vi "Read.vi"(7 "Delay (On)":bool=TRUE caption="Delay(ON)", 8 "error in (no error)":errorcluster, 9 "Termination Character (10)":u8=10, 10 "Byte Count (1024)":u32=1024, 11 "VISA resource name":refnum<visa-resource-name>) -> (0 "error out":errorcluster, 1 "Return Count":u32, 2 "Read Buffer":string, 3 "VISA resource name out":refnum<visa-resource-name>)   [LabVIEW 2009, in "DSO1K.lvlib"]
doc: "Reads the returns the data in read buffer."
uses:
  <instrlib>/DSO1K/DSO1K.lvlib
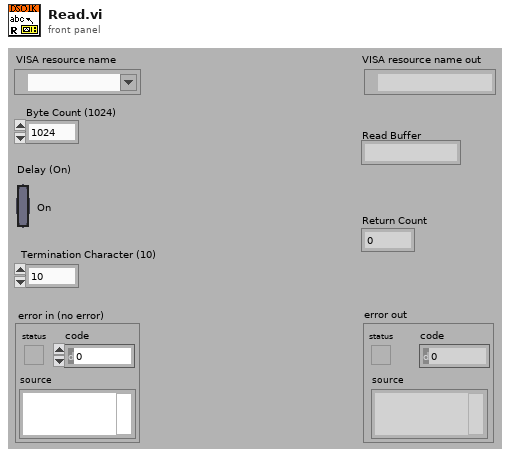
[diagram p1: front panel]
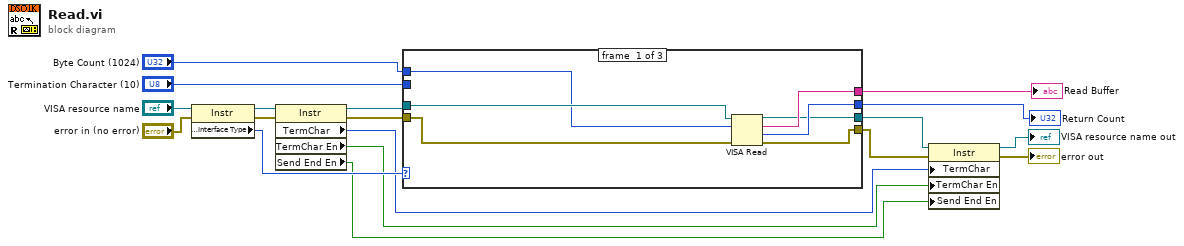
[diagram p0: block diagram]
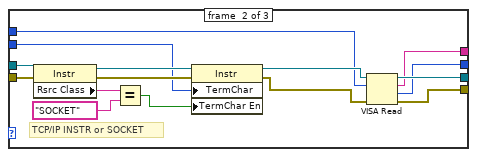
[diagram p2: hidden frame]
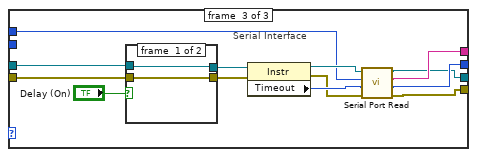
[diagram p3: hidden frame]
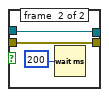
[diagram p4: hidden frame]
diagram:
  n1 = property class="Instr"(reference="VISA resource name", error in="error in (no error)") -> (reference out=w11:refnum<visa-resource-name>, error out=w13:errorcluster, "Interface Information:Interface Type"=w16:u16)
  n2 = property class="Instr"(reference=w11, error in=w13) -> (reference out=w10:refnum<visa-resource-name>, error out=w12:errorcluster, "TermChar"=w9:u8, "TermChar En"=w6:bool, "Send End En"=w8:bool)
  n3 = case shown="1..3, Default" w16 {
    tunnel: [w23 w31 w43] -> w3
    tunnel: w10 -> [w21 w40 w53]
    tunnel: [w22 w29 w46] -> w2
    tunnel: w12 -> [w20 w39 w50]
    tunnel: "Termination Character (10)" -> [_ w33 _]
    tunnel: [w24 w28 w44] -> w5
    tunnel: [w25 w27 w45] -> w4
    tunnel: "Byte Count (1024)" -> [w19 w26 w42]
    frame #0 {
      n4 = VISA Read(VISA resource name=w21, byte count=w19, error in (no error)=w20) -> (VISA resource name out=w23:refnum<visa-resource-name>, read buffer=w24:string, return count=w25:u32, error out=w22:errorcluster)
    }
    frame #1 {
      # "TCP/IP INSTR or SOCKET"
      n5 = property class="Instr"(reference=w40, error in=w39) -> (reference out=w35:refnum<visa-resource-name>, error out=w34:errorcluster, "Rsrc Class"=w38:string)
      n6 = Equal?(x=w38, y="SOCKET") -> (x = y?=w36:bool)
      n7 = property class="Instr"(reference=w35, error in=w34, "TermChar"=w33, "TermChar En"=w36) -> (reference out=w32:refnum<visa-resource-name>, error out=w30:errorcluster)
      n8 = VISA Read(VISA resource name=w32, byte count=w26, error in (no error)=w30) -> (VISA resource name out=w31:refnum<visa-resource-name>, read buffer=w28:string, return count=w27:u32, error out=w29:errorcluster)
    }
    frame #2 {
      # "Serial Interface"
      n9 = case shown="True" "Delay (On)" {
        tunnel: w53 -> [w55 w58]
        tunnel: [w55 w58] -> w52
        tunnel: [w54 w57] -> w51
        tunnel: w50 -> [w54 w57]
        frame #0 {
        }
        frame #1 {
          n10 = Wait (ms)(milliseconds to wait=u32 200) -> ()  [unwired: 1 out]
        }
      }
      n11 = property class="Instr"(reference=w52, error in=w51) -> (reference out=w48:refnum<visa-resource-name>, error out=w41:errorcluster, "Timeout"=w47:u32)
      n12 = call <instrlib>:"Serial Port Read.vi"("error in (no error)"=w41, "Timeout (2000ms)"=w47, "Byte Count"=w42, "VISA resource name"=w48) -> ("error out"=w46:errorcluster, "Return Count"=w45:u32, "Read Buffer"=w44:string, "VISA resource name out"=w43:refnum<visa-resource-name>)  [unwired: 4 in]
    }
  }
  "Return Count" <- w4
  "Read Buffer" <- w5
  n13 = property class="Instr"(reference=w3, error in=w2, "TermChar"=w9, "TermChar En"=w6, "Send End En"=w8) -> (reference out=→"VISA resource name out":refnum<visa-resource-name>, error out=→"error out":errorcluster)
